vi "practica 3.vi"() -> ()   [LabVIEW 2014]
panel:
  in  "stop (F)":bool
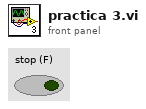
[diagram p1: front panel]
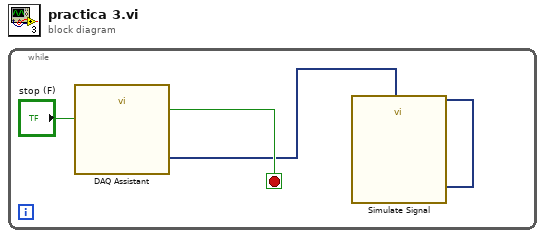
[diagram p0: block diagram]
diagram:
  n1 = while {
    stop <- w2 stop-if-true
    n2 = call "Simulate Signal"() -> ("Square"=w1:dynamicdata)  [unwired: 14 in, 1 out]
    n3 = call "DAQ Assistant"("data"=w1, "stop (F)"="stop (F)") -> ("stopped"=w2:bool)  [unwired: 15 in, 2 out]
  }
